vi "CorrectClimb.vi"(8 "BackEncoder":dbl, 9 "FrontEncoder":dbl, 10 "BackControl":dbl, 11 "FrontControl":dbl) -> (2 "BackOutput":dbl, 3 "FrontOutput":dbl)   [LabVIEW 2018]
uses:
  <vilib>/Rock Robotics/Network Tables/NT Read Number.vi
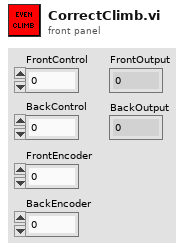
[diagram p1: front panel]
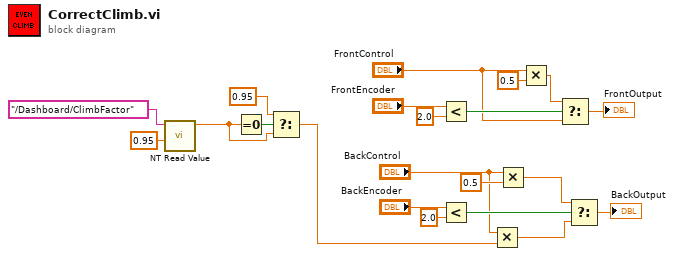
[diagram p0: block diagram]
diagram:
  n1 = call-poly <vilib>:"NT Read Value.vi"("Default Value"=0.95, "Name"="/Dashboard/ClimbFactor") -> ("Numeric"=w9:dbl)  [unwired: 8 in, 1 out]
  n2 = Equal To 0?(x=w9) -> (x = 0?=w10:bool)
  n3 = Select(t=0.95, s=w10, f=w9) -> (s? t:f=w3:dbl)
  n4 = Less?(x="FrontEncoder", y=2.0) -> (x < y?=w17:bool)
  n5 = Less?(x="BackEncoder", y=2.0) -> (x < y?=w20:bool)
  n6 = Multiply(x="BackControl", y=w3) -> (x*y=w1:dbl)
  n7 = Multiply(x="BackControl", y=0.5) -> (x*y=w5:dbl)
  n8 = Multiply(x="FrontControl", y=0.5) -> (x*y=w15:dbl)
  n9 = Select(t=w15, s=w17, f="FrontControl") -> (s? t:f=→"FrontOutput":dbl)
  n10 = Select(t=w5, s=w20, f=w1) -> (s? t:f=→"BackOutput":dbl)
